vi "Read Namespace Symbol Information.vi"(6 "Get all descendents?":bool, 8 "error in (no error)":errorcluster, 10 "Namespace":string, 11 "TwinCAT ADS in":refnum<class "TwinCAT ADS.lvclass">) -> (0 "error out":errorcluster, 1 "Symbols Information":T1[](array[typedef]) {"Type ID" items=["ADST_VOID"=0, "ADST_INT16"=2, "ADST_INT32"=3, "ADST_REAL32"=4, "ADST_REAL64"=5, "ADST_INT8"=16, "ADST_UINT8"=17, "ADST_UINT16"=18, "ADST_UINT32"=19, "ADST_INT64"=20, "ADST_UINT64"=21, "ADST_STRING"=30, "ADST_WSTRING"=31, "ADST_REAL80"=32, "ADST_BIT"=33, "ADST_MAXTYPES"=34, "ADST_BIGTYPE"=65]; "Type Category" items=["Unknown, None"=0, "Primitive"=1, "Alias"=2, "Enum"=3, "Array"=4, "Struct"=5, "FunctionBlock"=6, "Program"=7, "Function"=8, "SubRange"=9, "String"=10, "Bitset"=12, "Pointer"=13, "Union"=14, "Reference"=15, "Interface"=16]}, 3 "TwinCAT ADS out":refnum<class "TwinCAT ADS.lvclass">)   [LabVIEW 2018, in "TwinCAT ADS.lvclass"]
uses:
  TwinCAT ADS.lvclass
  Controls/Symbol Information.ctl
  TwinCAT.Ads
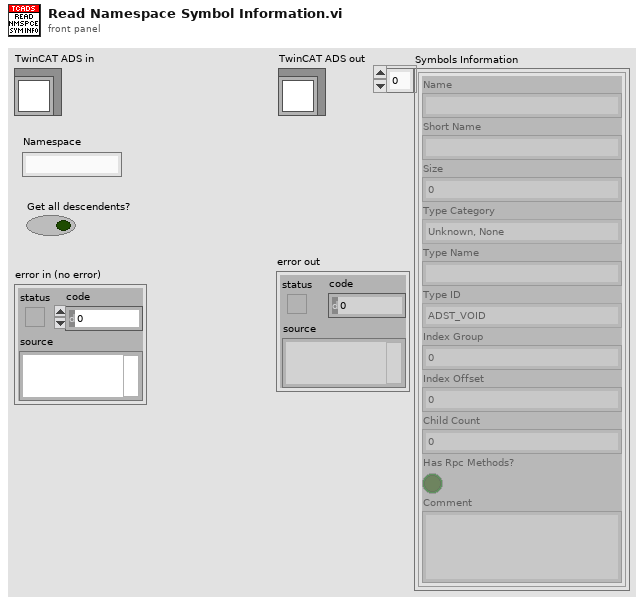
[diagram p1: front panel]
types:
  T1 = typedef "TwinCAT ADS.lvclass/Symbol Information.ctl" = cluster{"Name":string, "Short Name":string, "Size":i32, "Type Category":i32, "Type Name":string, "Type ID":i32, "Index Group":i64, "Index Offset":i64, "Child Count":i32, "Has Rpc Methods?":bool, "Comment":string}
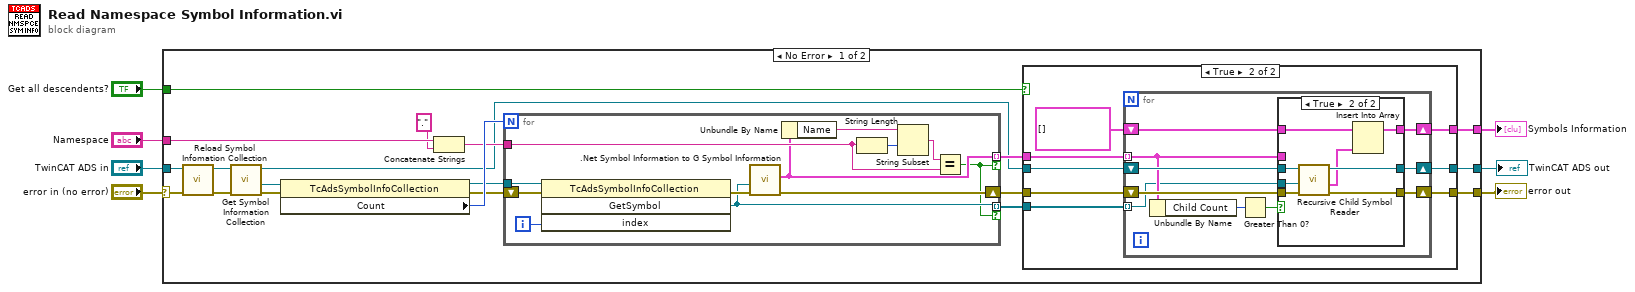
[diagram p0: block diagram]
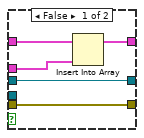
[diagram p3: hidden frame]
diagram:
  n1 = case shown="No Error" "error in (no error)" {
    selector: "error in (no error)" -> [w10 w75]
    tunnel: [w20 w75] -> w6
    tunnel: [w19 w74] -> w4
    tunnel: "TwinCAT ADS in" -> [w11 w74]
    tunnel: "Namespace" -> [w24 _]
    tunnel: [w17 _] -> w2
    tunnel: "Get all descendents?" -> [w16 _]
    frame No Error {
      n2 = call-dynamic "Reload Symbol Infomation Collection.vi"("error in (no error)"=w10, "TwinCAT ADS in"=w11) -> ("error out"=w8:errorcluster, "TwinCAT ADS out"=w9:refnum<class "TwinCAT ADS.lvclass">)  [unwired: 8 in]
      n3 = call-dynamic "Get Symbol Information Collection.vi"("error in (no error)"=w8, "TwinCAT ADS in"=w9) -> ("error out"=w14:errorcluster, "Symbol Info Collection"=w13:refnum<k24>, "TwinCAT ADS out"=w12:refnum<class "TwinCAT ADS.lvclass">)  [unwired: 7 in]
      n4 = property class="TcAdsSymbolInfoCollection"(reference=w13, error in=w14) -> (reference out=w25:refnum<k24>, error out=w26:errorcluster, "Count"=w27:i32)
      n5 = Concatenate Strings(w24, "." ("string")) -> (w22:string)
      n6 = for {
        N: w27 -> [_]
        tunnel: w25 -> [w73]
        shift-right: [w65] -> w21
        shift-left: w26 -> [w71]
        tunnel: w22 -> [w68]
        tunnel: [w64] -> w18 mode=indexing if=w62
        tunnel: [w63] -> w15 mode=indexing if=w62
        i -> [w72]
        n7 = invoke class="TcAdsSymbolInfoCollection" method="GetSymbol"(reference=w73, error in=w71, "index"=w72) -> (error out=w67:errorcluster, "GetSymbol"=w63:refnum<k24>)  [unwired: 1 in, 2 out]
        n8 = call ".Net Symbol Information to G Symbol Information.vi"(".NET ITcAdsSymbolInfo refnum"=w63, "error in (no error)"=w67) -> ("Symbol Information"=w64:T1, "error out"=w65:errorcluster)  [unwired: 6 in, 1 out]
        n9 = Unbundle By Name(w64) -> ("Name"=w66:string)
        n10 = String Length(string=w68) -> (length=w70:i32)
        n11 = String Subset(string=w66, length (rest)=w70) -> (substring=w69:string)  [unwired: 1 in]
        n12 = Equal?(x=w69, y=w68) -> (x = y?=w62:bool)
      }
      n13 = case shown="True" w16 {
        tunnel: w21 -> [w30 w38]
        tunnel: [w30 w37] -> w20
        tunnel: [w28 w36] -> w19
        tunnel: w12 -> [w28 w35]
        tunnel: w18 -> [w29 w34]
        tunnel: [w29 w33] -> w17
        tunnel: w15 -> [_ w31]
        frame False {
        }
        frame True {
          n14 = for {
            shift-right: [w48] -> w37
            shift-left: w38 -> [w42]
            shift-right: [w47] -> w36
            shift-left: w35 -> [w46]
            tunnel: w34 -> [w40] mode=indexing
            shift-right: [w43] -> w33
            shift-left: T1[] [] -> [w44]
            tunnel: w31 -> [w39] mode=indexing
            n15 = Unbundle By Name(w40) -> ("Child Count"=w41:i32)
            n16 = Greater Than 0?(x=w41) -> (x > 0?=w45:bool)
            n17 = case shown="True" w45 {
              tunnel: w42 -> [w53 w59]
              tunnel: [w53 w55] -> w48
              tunnel: [w52 w56] -> w47
              tunnel: w46 -> [w52 w57]
              tunnel: w40 -> [w49 _]
              tunnel: w44 -> [w51 w61]
              tunnel: [w50 w60] -> w43
              tunnel: w39 -> [_ w58]
              frame False {
                n18 = Insert Into Array(array=w51, new element=w49) -> (w50:T1[])  [unwired: 1 in]
              }
              frame True {
                n19 = call "Recursive Child Symbol Reader.vi"("error in (no error)"=w59, ".NET TcAdsSymbolInfo"=w58, "TwinCAT ADS in"=w57) -> ("error out"=w55:errorcluster, "Symbols Information"=w54:T1[], "TwinCAT ADS out"=w56:refnum<class "TwinCAT ADS.lvclass">)  [unwired: 6 in]
                n20 = Insert Into Array(array=w61, new element=w54) -> (w60:T1[])  [unwired: 1 in]
              }
            }
          }
        }
      }
    }
    frame Error {
    }
  }
  "error out" <- w6
  "TwinCAT ADS out" <- w4
  "Symbols Information" <- w2
